vi "Basic DVR Qs.vi"() -> ()   [LabVIEW 2021, in "Q Async.lvlib"]
uses:
  Q Async.lvlib
panel:
  in  "Numeric":i32=3
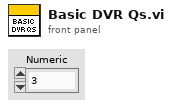
[diagram p1: front panel]
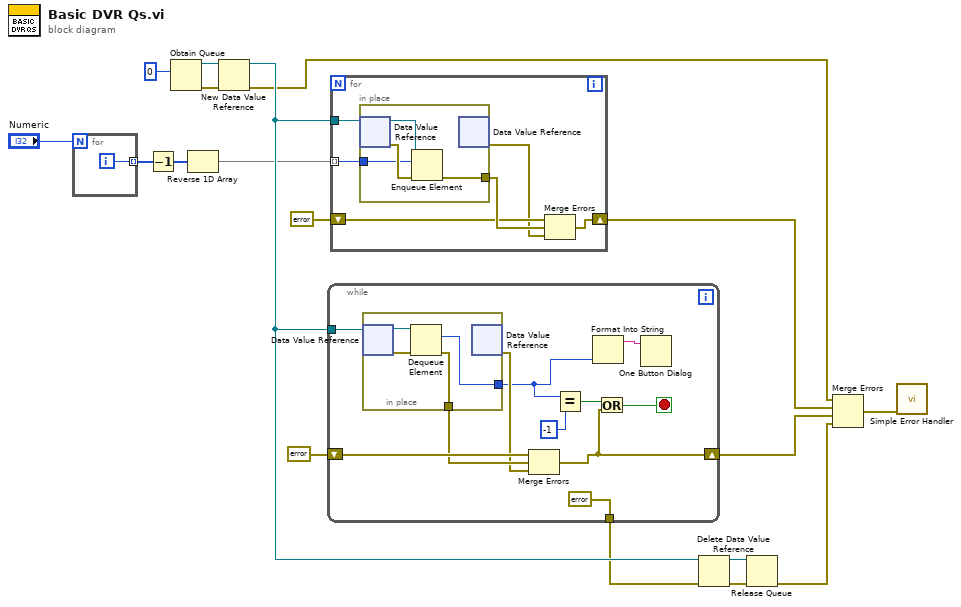
[diagram p0: block diagram]
diagram:
  n1 = for {
    N: "Numeric" -> [_]
    tunnel: [w19] -> w17 mode=indexing
    i -> [w19]
  }
  n2 = Decrement(x=w17) -> (x-1=w18:i32[])
  n3 = Obtain Queue(element data type=0) -> (queue out=w15:refnum<queue>, error out=w8:errorcluster)  [unwired: 4 in, 1 out]
  n4 = Reverse 1D Array(array=w18) -> (reversed array=w12:i32[])
  n5 = New Data Value Reference(data value=w15, error in=w8) -> (data value reference=w13:refnum<data-value>, error out=w1:errorcluster)
  n6 = while {
    tunnel: w13 -> [w28]
    tunnel: [errorcluster {"status"=FALSE, "code"=0, "source"=""} ("error in (no error)")] -> w11
    shift-right: [w20] -> w4
    shift-left: errorcluster {"status"=FALSE, "code"=0, "source"=""} ("error IO") -> [w26]
    stop <- w21 stop-if-true
    n7 = in-place {
      in-place-border: [w34] -> w22
      in-place-border: [w31] -> w25
      n8 = in-place-dvr #1(w28) -> (w33:refnum<queue>, w32:errorcluster)
      n9 = Dequeue Element(queue=w33, error in (no error)=w32) -> (element=w34:i32, error out=w31:errorcluster)  [unwired: 1 in, 2 out]
      n10 = in-place-dvr #1() -> (w24:errorcluster)  [unwired: 1 in, 1 out]
    }
    n11 = Merge Errors(w26, w25, w24) -> (w20:errorcluster)
    n12 = Equal?(x=w22, y=-1) -> (x = y?=w30:bool)
    n13 = Format Into String(w22) -> (resulting string=w23:string)  [unwired: 3 in, 1 out]
    n14 = Or(x=w30, y=w20) -> (x .or. y?=w21:bool)
    n15 = One Button Dialog(message=w23) -> ()  [unwired: 1 in, 1 out]
  }
  n16 = for {
    tunnel: w13 -> [w40]
    tunnel: w12 -> [w39] mode=indexing
    shift-right: [w37] -> w5
    shift-left: errorcluster {"status"=FALSE, "code"=0, "source"=""} ("error out") -> [w36]
    n17 = in-place {
      in-place-border: w39 -> [w41]
      in-place-border: [w42] -> w38
      n18 = in-place-dvr #2(w40) -> (w44:refnum<queue>, w43:errorcluster)
      n19 = Enqueue Element(queue=w44, element=w41, error in (no error)=w43) -> (error out=w42:errorcluster)  [unwired: 1 in, 2 out]
      n20 = in-place-dvr #2() -> (w35:errorcluster)  [unwired: 1 in, 1 out]
    }
    n21 = Merge Errors(w36, w38, w35) -> (w37:errorcluster)
  }
  n22 = Delete Data Value Reference(data value reference=w13, error in=w11) -> (data value=w10:refnum<queue>, error out=w9:errorcluster)
  n23 = Release Queue(queue=w10, error in (no error)=w9) -> (error out=w3:errorcluster)  [unwired: 1 in, 2 out]
  n24 = Merge Errors(w1, w5, w4, w3) -> (w2:errorcluster)
  n25 = call <vilib>:"Simple Error Handler.vi"("error in (no error)"=w2) -> ()  [unwired: 4 in, 5 out]
